vi "__anritsu_setup.vi"(0 "Center Freq (Hz)":dbl, 1 "Points":i32, 2 "address":string="192.168.0.6", 5 "Span (Hz)":dbl, 7 "RBW (Hz)":dbl, 9 "VBW (Hz)":dbl, 11 "error in (no error)":errorcluster) -> (4 "Anritsu command":string, 15 "error out":errorcluster)   [LabVIEW 2013]
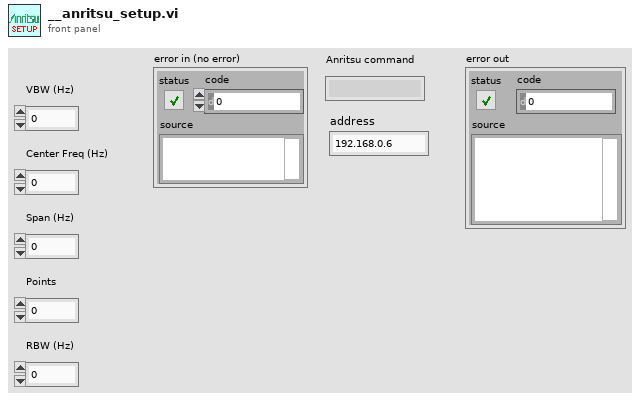
[diagram p1: front panel]
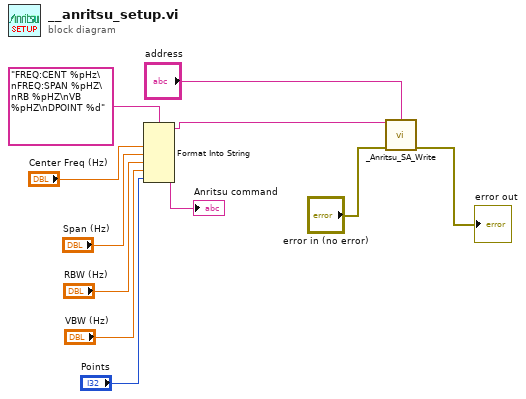
[diagram p0: block diagram]
diagram:
  n1 = Format Into String(format string="FREQ:CENT %pHz\nFREQ:SPAN %pHZ\nRB %pHZ\nVB %pHZ\nDPOINT %d" ("Comand"), "Center Freq (Hz)", "Span (Hz)", "RBW (Hz)", "VBW (Hz)", "Points") -> (resulting string=w5:string)  [unwired: 2 in, 1 out]
  "Anritsu command" <- w5
  n2 = call "_Anritsu_SA_Write.vi"("Comand"=w5, "address"="address", "error in (no error)"="error in (no error)") -> ("error out"=→"error out":errorcluster)  [unwired: 12 in]
